vi "DAQmx Control Digital Output (SubVI).vi"(0 "Digital Output Module Configure":T1={"Module Type"=enum."SCXI", "DAQ #"=1, "Module #"=4}, 3 "Relay Control":bool[](array[boolean]), 9 "E-STOP Input":bool) -> (14 "Task OUT":refnum<k21>, 19 "Error OUT":errorcluster)   [LabVIEW 2009]
uses:
  <vilib>/DAQmx/create/channels.llb/DAQmx Create Channel (DO-Digital Output).vi
  <vilib>/DAQmx/write.llb/DAQmx Write (Digital 1D Bool NChan 1Samp 1Line).vi
  C:/Program Files/National Instruments/LabVIEW 2009/resource/objmgr/daqmx.rc
panel:
  # "Created by Blake Otting\n3/29/2010"
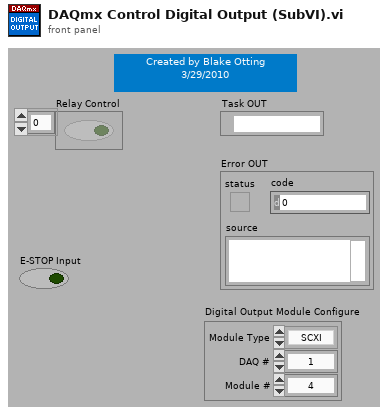
[diagram p1: front panel]
types:
  T1 = cluster{"Module Type":enum16{"CDAQ", "SCXI"}, "DAQ #":i32, "Module #":i32}
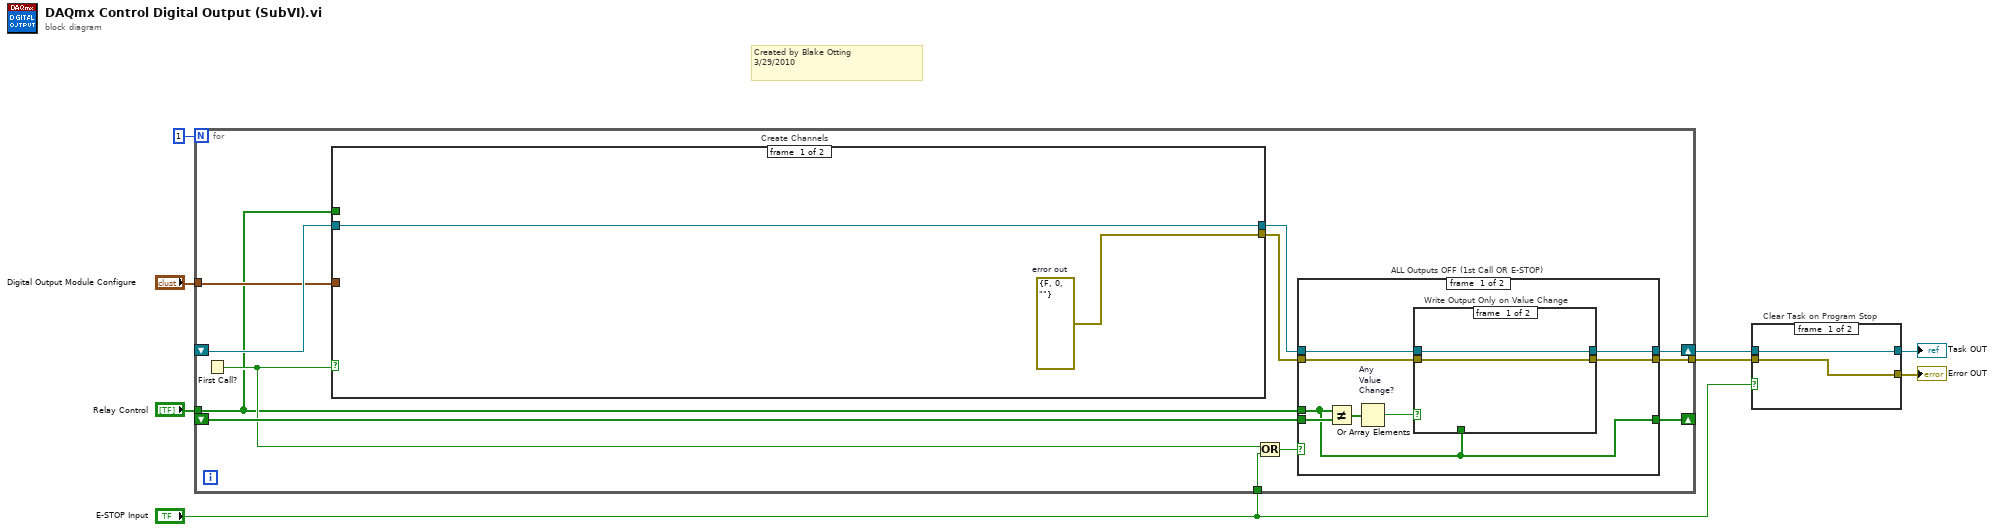
[diagram p0: block diagram]
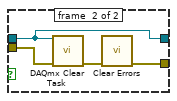
[diagram p2: hidden frame]
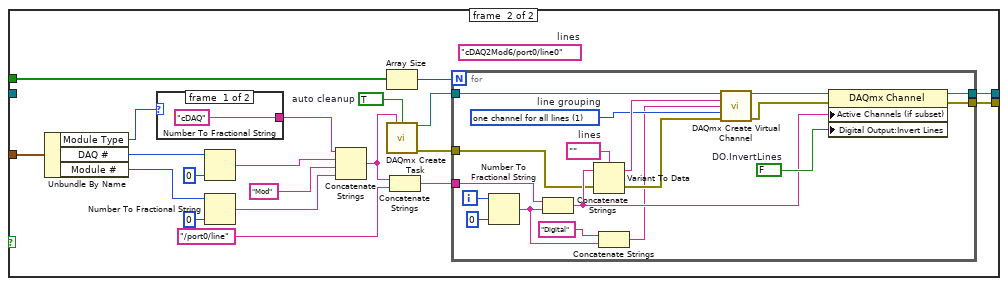
[diagram p3: hidden frame]
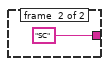
[diagram p4: hidden frame]
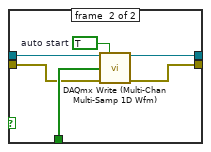
[diagram p5: hidden frame]
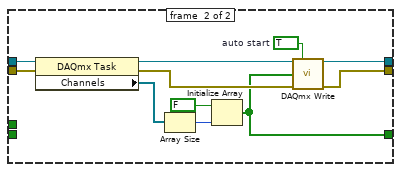
[diagram p6: hidden frame]
diagram:
  # "Created by Blake Otting\n3/29/2010"
  n1 = for {
    N: 1 -> [_]
    tunnel: [w20] -> w5
    shift-right: [w19] -> _
    shift-left: _ -> [w18]
    tunnel: "Relay Control" -> [w9]
    tunnel: "E-STOP Input" -> [w16]
    shift-right: [w15] -> w2
    shift-left: _ -> [w13]
    tunnel: "Digital Output Module Configure" -> [w11]
    n2 = First Call?() -> (First Call?: T/F=w10:bool)
    n3 = case "Create Channels" shown="False" w10 {
      tunnel: w11 -> [_ w35]
      tunnel: [w21 w34] -> w14
      tunnel: [w22 w33] -> w12
      tunnel: w13 -> [w21 _]
      tunnel: w9 -> [_ w25]
      frame #0 {
        w22 = errorcluster {"status"=FALSE, "code"=0, "source"=""}  # error out
      }
      frame #1 {
        (unwired) "cDAQ2Mod6/port0/line0"  # lines
        w30 = TRUE  # auto cleanup
        n4 = Unbundle By Name(w35) -> ("Module Type"=w23:enum16{"CDAQ", "SCXI"}, "DAQ #"=w37:i32, "Module #"=w36:i32)
        n5 = case shown="\"CDAQ\", Default" w23 {
          tunnel: ["cDAQ" ("physical channel") "SC" ("physical channel")] -> w24
          frame #0 {
          }
          frame #1 {
          }
        }
        n6 = Number To Fractional String(number=w37, precision (6)=i16 0) -> (F-format string=w40:string)  [unwired: 2 in]
        n7 = Number To Fractional String(number=w36, precision (6)=i16 0) -> (F-format string=w38:string)  [unwired: 2 in]
        n8 = Concatenate Strings(w24, w40, "Mod" ("physical channel"), w38) -> (w28:string)
        n9 = Array Size(array=w25) -> (size(s)=w32:i32)
        n10 = call <vilib>:"DAQmx Create Task.vi"("new task name"=w28, "auto cleanup"=w30) -> ("task out"=w29:refnum<k21>, "error out"=w31:errorcluster)  [unwired: 12 in]
        n11 = Concatenate Strings(w28, "/port0/line" ("physical channel")) -> (w26:string)
        n12 = for {
          N: w32 -> [_]
          tunnel: w26 -> [w53]
          tunnel: w31 -> [w51]
          tunnel: [w50] -> w34
          tunnel: [w49] -> w33
          tunnel: w29 -> [w48]
          i -> [w54]
          w56 = 1 items=["one channel for each line", "one channel for all lines"]  # line grouping
          w57 = FALSE  # DO.InvertLines
          w62 = tag ""  # lines
          n13 = Number To Fractional String(number=w54, precision (6)=i16 0) -> (F-format string=w46:string)  [unwired: 2 in]
          n14 = Concatenate Strings(w53, w46) -> (w52:string)
          n15 = Variant To Data(error in=w51, Variant=w52, type=w62) -> (error out=w60:errorcluster, data=w61:tag)
          n16 = Concatenate Strings("Digital" ("string"), w46) -> (w45:string)
          n17 = call-poly <vilib>:"DAQmx Create Virtual Channel.vi"("task in"=w48, "lines"=w61, "name to assign"=w45, "line grouping"=w56, "error in"=w60) -> ("task out"=w59:refnum<k21>, "error out"=w58:errorcluster)  [unwired: 9 in]
          n18 = property class="DAQmx Channel"(reference=w59, error in=w58, "Active Channels (if subset)"=w52, "Digital Output:Invert Lines"=w57) -> (reference out=w50:refnum<k21>, error out=w49:errorcluster)
        }
      }
    }
    n19 = Or(x=w10, y=w16) -> (x .or. y?=w17:bool)
    n20 = case "ALL Outputs OFF (1st Call OR E-STOP)" shown="False" w17 {
      tunnel: w14 -> [w70 w87]
      tunnel: w12 -> [w67 w86]
      tunnel: [w69 w81] -> w15
      tunnel: [w68 w82] -> w20
      tunnel: [w64 w79] -> w19
      tunnel: w18 -> [w66 _]
      tunnel: w9 -> [w64 _]
      frame #0 {
        n21 = Not Equal?(x=w64, y=w66) -> (x != y?=w65:bool[])
        n22 = Or Array Elements "Any\nValue\nChange?"(Boolean array=w65) -> (logical OR=w63:bool)
        n23 = case "Write Output Only on Value Change" shown="True" w63 {
          tunnel: w70 -> [w72 w78]
          tunnel: [w72 w77] -> w69
          tunnel: [w71 w75] -> w68
          tunnel: w64 -> [_ w74]
          tunnel: w67 -> [w71 w73]
          frame #0 {
          }
          frame #1 {
            w76 = TRUE  # auto start
            n24 = call-poly "DAQmx Write (Multi-Chan Multi-Samp 1D Wfm).vi"("task/channels in"=w78, "auto start"=w76, "data"=w74, "error in"=w73) -> ("task out"=w77:refnum<k21>, "error out"=w75:errorcluster)  [unwired: 9 in, 1 out]
          }
        }
      }
      frame #1 {
        w80 = TRUE  # auto start
        n25 = property class="DAQmx Task"(reference=w87, error in=w86) -> (reference out=w85:refnum<k21>, error out=w84:errorcluster, "Channels"=w89:refnum<k21>[])
        n26 = Array Size(array=w89) -> (size(s)=w88:i32)
        n27 = Initialize Array(FALSE ("element"), w88) -> (w79:bool[])
        n28 = call-poly <vilib>:"DAQmx Write.vi"("task/channels in"=w85, "auto start"=w80, "data"=w79, "error in"=w84) -> ("task out"=w81:refnum<k21>, "error out"=w82:errorcluster)  [unwired: 9 in, 1 out]
      }
    }
  }
  n29 = case "Clear Task on Program Stop" shown="True" "E-STOP Input" {
    tunnel: w5 -> [w90 w94]
    tunnel: [w90 w93] -> w7
    tunnel: w2 -> [w91 w92]
    tunnel: [w91 w92] -> w6
    frame #0 {
    }
    frame #1 {
      n30 = call <vilib>:"DAQmx Clear Task.vi"("task in"=w92, "error in"=w94) -> ("error out"=w95:errorcluster)  [unwired: 13 in]
      n31 = call <vilib>:"Clear Errors.vi"("error in (no error)"=w95) -> ("error out"=w93:errorcluster)  [unwired: 6 in]
    }
  }
  "Task OUT" <- w6
  "Error OUT" <- w7
